vi "Quad Encoder - Host.vi"() -> ()   [LabVIEW 8.6]
doc: "I. Description:\nThis is the Host VI for the Quadrature Encoder Personality. The purpose of this VI is to read 6 Quadrature Encoder Inputs and control 2 Quadrature Encoder Outputs. DIO lines 0 thru 5 on Connector 0 are configured as Quadrature Encoder Inputs. DIO lines 6 thru 7 on Connector 0 are configured as Quadrature Encoder Outputs. This VI also utilizes the DIO lines on connector 1 as static digital inputs and on connector 2 as static digital outputs.\n\n\nII. Instructions for Running:\n1. Select the Resource Name for the target R Series board.\n2. Specify the Frequency and Duty cycle for the desired output channels.\n3. Run the VI\n4. Toggle the Digital Output lines and PWM Output lines as needed.\n\nIII. Steps: \n1. Define the Resource Name for the target R Series board and open a reference to it.\n2. Initialize the Inputs/ Outputs on the R Series board. \n3. Call the FreqtoTicks VI to convert the Frequency to the corresponding Ticks for output channels.\n4. Call the Read/ Write Control to read the position of the encoder inputs and to write the frequency and direction for the encoder outputs.\n5. Call the PulsetoFreq VI to convert the High and Low Time in Ticks to the corresponding Frequency and Duty Cycle for input channels.\n6. Call Close FPGA VI Reference VI to close the reference to the R Series board. \n7. Use the popup dialog box to display an error if any.\n\nIV. I/O Connections Overview:\nQuad Enc Inputs DIO Lines 00-11 (Connector 0)\nQuad Enc Outputs DIO Lines 6-7 (Connector 0)\nDigital Outputs DIO Lines 00-39 (Connector 1)\nDigital Inputs DIO Lines 00-39 (Connector 2)"
uses:
  <vilib>/rvi/interface/nirviOpenFPGA/nirviOpenFPGA.xnode
  <vilib>/rvi/interface/nirviReadWriteControl/nirviReadWriteControl.xnode
  <vilib>/rvi/interface/nirviCloseFPGA/nirviCloseFPGA.xnode
  FPGA Bitfiles/Quadrature Encoder PCI-7811.lvbit
  <vilib>/userdefined/High Color/nirio_resource_hc.ctl
panel:
  in  "Quadrature Encoder Type":T1(ring)
  in  "Stop Button":bool
  in  "Frequency (Hz) - Quad 7":dbl
  in  "Frequency (Hz) - Quad 6":dbl
  in  "Direction - Quad 7":bool
  in  "Direction - Quad 6":bool
  in  "Reset - Quad 5":bool
  in  "Reset - Quad 4":bool
  in  "Reset - Quad 3":bool
  in  "Reset - Quad 2":bool
  in  "Reset - Quad 1":bool
  in  "Reset - Quad 0":bool
  out "Encoder Position - Quad 3":dbl
  out "Encoder Position - Quad 4":dbl
  out "Encoder Position - Quad 5":dbl
  out "Encoder Position - Quad 2":dbl
  out "Encoder Position - Quad 1":dbl
  out "Encoder Position - Quad 0":dbl
  in  "DIOPORT0":bool[](array[boolean]) caption="DIOPORT 0"
  in  "DIOPORT1":bool[](array[boolean]) caption="DIOPORT 1"
  in  "DIOPORT2":bool[](array[boolean]) caption="DIOPORT 2"
  in  "DIOPORT3":bool[](array[boolean]) caption="DIOPORT 3"
  in  "DIOPORT4":bool[](array[boolean]) caption="DIOPORT 4"
  out "DIOPORT0":bool[](array[boolean]) caption="DIOPORT 0"
  out "DIOPORT1":bool[](array[boolean]) caption="DIOPORT 1"
  out "DIOPORT2":bool[](array[boolean]) caption="DIOPORT 2"
  out "DIOPORT3":bool[](array[boolean]) caption="DIOPORT 3"
  out "DIOPORT4":bool[](array[boolean]) caption="DIOPORT 4"
  in  "Resource Name":T2
  in  "Steps per Revolution":dbl
  # "For instructions, select Help>>Show Context Help"
  # "Quadrature Encoder Inputs (Connector 0)"
  # "Digital Inputs (Connector 2)"
  # "7"
  # "5"
  # "4"
  # "3"
  # "2"
  # "1"
  # "0"
  # "6"
  # "Channel 0"
  # "Channel 1"
  # "Channel 2"
  # "Channel 3"
  # "Digital Outputs (Connector 1)"
  # "7"
  # "6"
  # "5"
  # "4"
  # "3"
  # "2"
  # "1"
  # "0"
  # "Channel 4"
  # "Channel 5"
  # "Quadrature Encoder Outputs (Connector 0)"
  # "Channel 6"
  # "Channel 7"
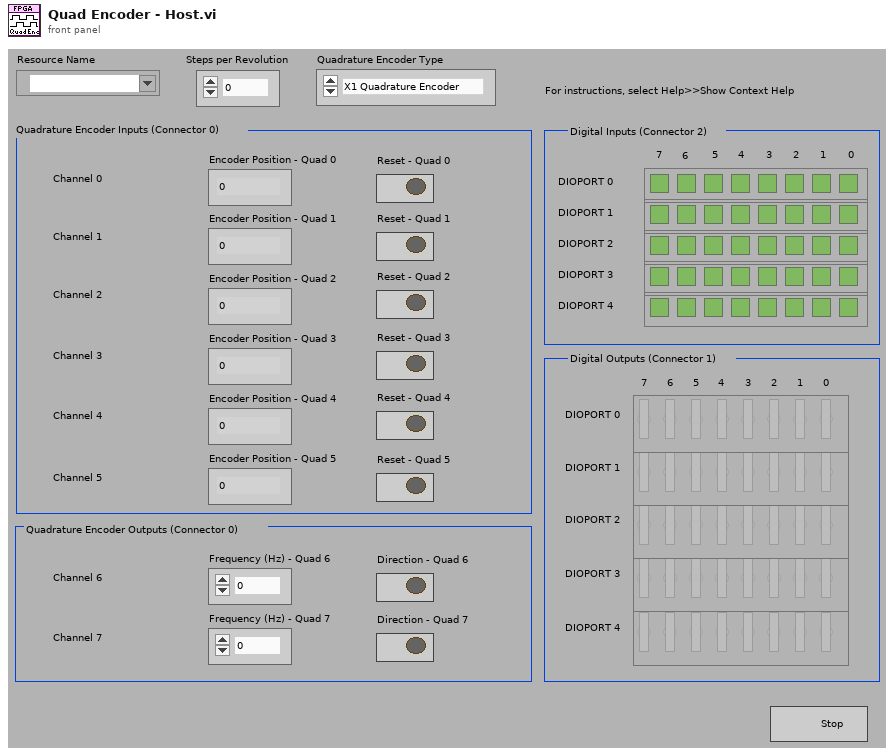
[diagram p1: front panel]
types:
  T1 = enum16{"X1 Quadrature Encoder", "X2 Quadrature Encoder", "X4 Quadrature Encoder"}
  T2 = typedef "nirio_resource_hc.ctl" = tag
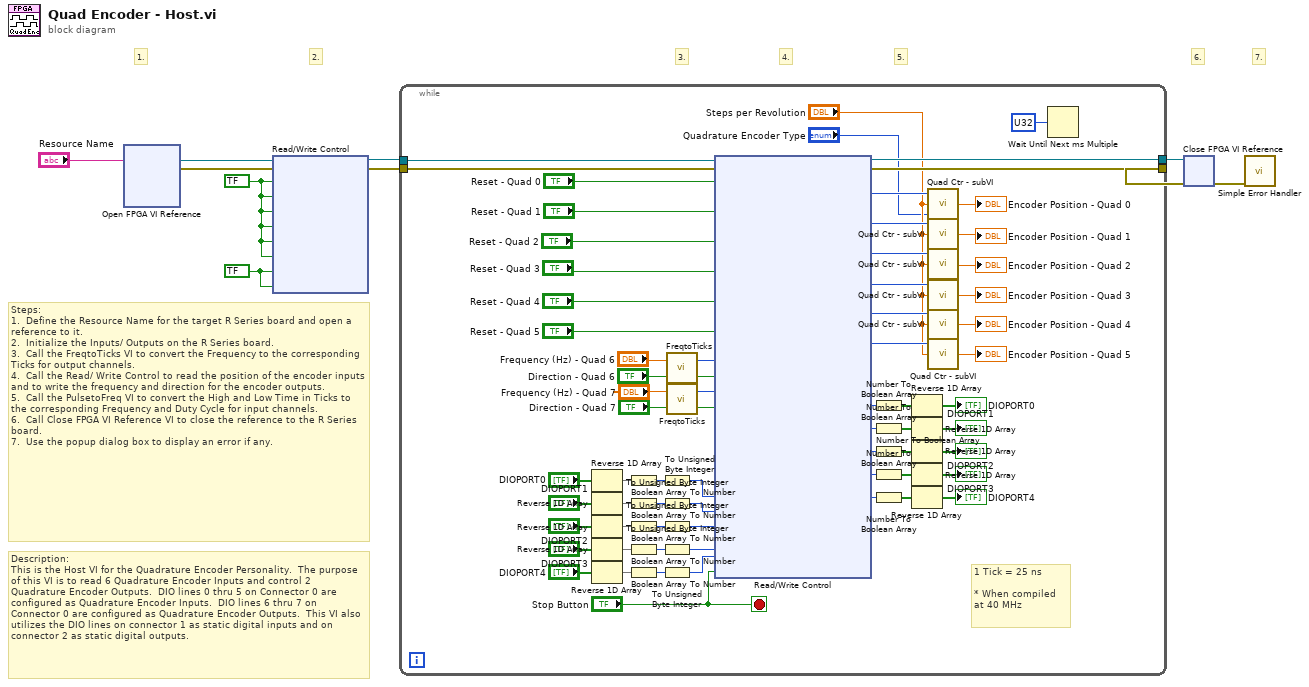
[diagram p0: block diagram]
diagram:
  w2 = bool ? ("Input - Quad 0")
  w3 = bool ? ("Input - Quad 0")
  # "6."
  # "4."
  # "7."
  # "5."
  # "3."
  # "2."
  # "1."
  # "Description:\nThis is the Host VI for the Quadrature Encoder Personality.  The purpose of this VI is to read 6 Quadrature Encoder Inputs and control 2 Quadrature Encoder Outputs.  DIO lines 0 thru 5 on Connector 0 are configured as Quadrature Encoder Inputs.  DIO lines 6 thru 7 on Connector 0 are configured as Quadrature Encoder Outputs.  This VI also utilizes the DIO lines on connector 1 as static digital inputs and on connector 2 as static digital outputs."
  # "Steps: \n1.  Define the Resource Name for the target R Series board and open a reference to it.\n2.  Initialize the Inputs/ Outputs on the R Series board.  \n3.  Call the FreqtoTicks VI to convert the Frequency to the corresponding Ticks for output channels.\n4.  Call the Read/ Write Control to read the position of the encoder inputs and to write the frequency and direction for the encoder outputs.\n5.  Call the PulsetoFreq VI to convert the High and Low Time in Ticks to the corresponding Frequency and Duty Cycle for input channels.\n6.  Call Close FPGA VI Reference VI to close the reference to the R Series board. \n7.  Use the popup dialog box to display an error if any."
  n1 = xnode "Open FPGA VI Reference"("resource name"="Resource Name") -> ("FPGA VI Reference Out"=w7:refnum<k20>, "error out"=w6:errorcluster)  [unwired: 1 in]
  n2 = xnode "Read/Write Control"("FPGA VI Reference In"=w7, "error in"=w6, "Input - Quad 0"=w3, "Input - Quad 1"=w3, "Input - Quad 2"=w3, "Input - Quad 3"=w3, "Input - Quad 4"=w3, "Input - Quad 5"=w3, "Input - Quad 6"=w2, "Input - Quad 7"=w2) -> ("FPGA VI Reference Out"=w5:refnum<k20>, "error out"=w4:errorcluster)
  n3 = while {
    tunnel: [w79] -> w10
    tunnel: [w78] -> w9
    tunnel: w5 -> [w76]
    tunnel: w4 -> [w75]
    stop <- "Stop Button" stop-if-true
    # "1 Tick = 25 ns\n\n* When compiled at 40 MHz"
    n4 = Reverse 1D Array(array="DIOPORT0") -> (reversed array=w62:bool[])
    n5 = Reverse 1D Array(array="DIOPORT1") -> (reversed array=w54:bool[])
    n6 = Reverse 1D Array(array="DIOPORT2") -> (reversed array=w55:bool[])
    n7 = Reverse 1D Array(array="DIOPORT3") -> (reversed array=w56:bool[])
    n8 = Reverse 1D Array(array="DIOPORT4") -> (reversed array=w57:bool[])
    n9 = Boolean Array To Number(Boolean array=w62) -> (number=w63:u32)
    n10 = Boolean Array To Number(Boolean array=w54) -> (number=w58:u32)
    n11 = Boolean Array To Number(Boolean array=w55) -> (number=w59:u32)
    n12 = Boolean Array To Number(Boolean array=w56) -> (number=w60:u32)
    n13 = Boolean Array To Number(Boolean array=w57) -> (number=w61:u32)
    n14 = To Unsigned Byte Integer(number=w63) -> (unsigned 8bit integer=w31:u8)
    n15 = To Unsigned Byte Integer(number=w58) -> (unsigned 8bit integer=w32:u8)
    n16 = To Unsigned Byte Integer(number=w59) -> (unsigned 8bit integer=w33:u8)
    n17 = To Unsigned Byte Integer(number=w60) -> (unsigned 8bit integer=w30:u8)
    n18 = To Unsigned Byte Integer(number=w61) -> (unsigned 8bit integer=w29:u8)
    n19 = call "FreqtoTicks.vi"("Boolean"="Direction - Quad 6", "Frequency"="Frequency (Hz) - Quad 6") -> ("Boolean 2"=w67:bool, "Numeric"=w68:u32)
    n20 = call "FreqtoTicks.vi"("Boolean"="Direction - Quad 7", "Frequency"="Frequency (Hz) - Quad 7") -> ("Boolean 2"=w65:bool, "Numeric"=w66:u32)
    n21 = xnode "Read/Write Control"("FPGA VI Reference In"=w76, "error in"=w75, "Reset - Quad 0"="Reset - Quad 0", "Reset - Quad 1"="Reset - Quad 1", "Reset - Quad 2"="Reset - Quad 2", "Reset - Quad 3"="Reset - Quad 3", "Reset - Quad 4"="Reset - Quad 4", "Reset - Quad 5"="Reset - Quad 5", "Period (Ticks) - Quad 6"=w68, "Direction - Quad 6"=w67, "Period (Ticks) - Quad 7"=w66, "Direction - Quad 7"=w65, "Connector 2 DIO Port 0"=w31, "Connector 2 DIO Port 1"=w32, "Connector 2 DIO Port 2"=w33, "Connector 2 DIO Port 3"=w30, "Connector 2 DIO Port 4"=w29, "stop"="Stop Button") -> ("FPGA VI Reference Out"=w79:refnum<k20>, "error out"=w78:errorcluster, "Encoder Position - Quad 0"=w74:i32, "Encoder Position - Quad 1"=w69:i32, "Encoder Position - Quad 2"=w70:i32, "Encoder Position - Quad 3"=w71:i32, "Encoder Position - Quad 4"=w72:i32, "Encoder Position - Quad 5"=w73:i32, "Connector 1 DIO Port 0"=w36:u8, "Connector 1 DIO Port 1"=w37:u8, "Connector 1 DIO Port 2"=w38:u8, "Connector 1 DIO Port 3"=w35:u8, "Connector 1 DIO Port 4"=w34:u8)
    n22 = Number To Boolean Array(number=w36) -> (Boolean array=w53:bool[])
    n23 = Number To Boolean Array(number=w37) -> (Boolean array=w52:bool[])
    n24 = Number To Boolean Array(number=w38) -> (Boolean array=w51:bool[])
    n25 = Number To Boolean Array(number=w35) -> (Boolean array=w50:bool[])
    n26 = Number To Boolean Array(number=w34) -> (Boolean array=w49:bool[])
    n27 = Reverse 1D Array(array=w53) -> (reversed array=→"DIOPORT0":bool[])
    n28 = Reverse 1D Array(array=w52) -> (reversed array=→"DIOPORT1":bool[])
    n29 = Reverse 1D Array(array=w51) -> (reversed array=→"DIOPORT2":bool[])
    n30 = Reverse 1D Array(array=w50) -> (reversed array=→"DIOPORT3":bool[])
    n31 = Reverse 1D Array(array=w49) -> (reversed array=→"DIOPORT4":bool[])
    n32 = call "Quad Ctr - subVI.vi"("Quadrature Encoder Type"="Quadrature Encoder Type", "Steps per Revolution"="Steps per Revolution", "16 bit Position 4"=w74) -> ("Position (Degrees)"=→"Encoder Position - Quad 0":dbl)
    n33 = call "Quad Ctr - subVI.vi"("Steps per Revolution"="Steps per Revolution", "16 bit Position 4"=w69) -> ("Position (Degrees)"=→"Encoder Position - Quad 1":dbl)  [unwired: 1 in]
    n34 = call "Quad Ctr - subVI.vi"("Steps per Revolution"="Steps per Revolution", "16 bit Position 4"=w70) -> ("Position (Degrees)"=→"Encoder Position - Quad 2":dbl)  [unwired: 1 in]
    n35 = call "Quad Ctr - subVI.vi"("Steps per Revolution"="Steps per Revolution", "16 bit Position 4"=w71) -> ("Position (Degrees)"=→"Encoder Position - Quad 3":dbl)  [unwired: 1 in]
    n36 = call "Quad Ctr - subVI.vi"("Steps per Revolution"="Steps per Revolution", "16 bit Position 4"=w72) -> ("Position (Degrees)"=→"Encoder Position - Quad 4":dbl)  [unwired: 1 in]
    n37 = call "Quad Ctr - subVI.vi"("Steps per Revolution"="Steps per Revolution", "16 bit Position 4"=w73) -> ("Position (Degrees)"=→"Encoder Position - Quad 5":dbl)  [unwired: 1 in]
    n38 = Wait Until Next ms Multiple(millisecond multiple=u32 ?) -> ()  [unwired: 1 out]
  }
  n39 = xnode "Close FPGA VI Reference"("FPGA VI Reference In"=w10, "error in"=w9) -> ("error out"=w1:errorcluster)
  n40 = call <vilib>:"Simple Error Handler.vi"("error in (no error)"=w1) -> ()  [unwired: 4 in, 5 out]
